vi "2D barcode scanning.vi"() -> ()   [LabVIEW 2015]
panel:
  in  "Find Max and Min":bool
  out "Optical Angle Waveform Graph":dynamicdata(graph)
  out "PSD Waveform Graph":dynamicdata(graph)
  out "Photodiode Waveform Graph":dynamicdata(graph)
  out "XY Graph":cluster{"Y":dbl[], "Y":dbl[]}[](graph)
  out "Offset Voltage":dbl
  out "Optical Angle":dynamicdata(graph)
  out "Min. Volt":dbl
  out "Max. Volt":dbl
  out "PSD Voltage":dbl format="%_15g"
  out "PSD (voltage)":dynamicdata(graph)
  out "Photodiode Waveform Chart (V)":dynamicdata(graph)
  out "Photodiode":dbl
  in  "stop (F)":bool
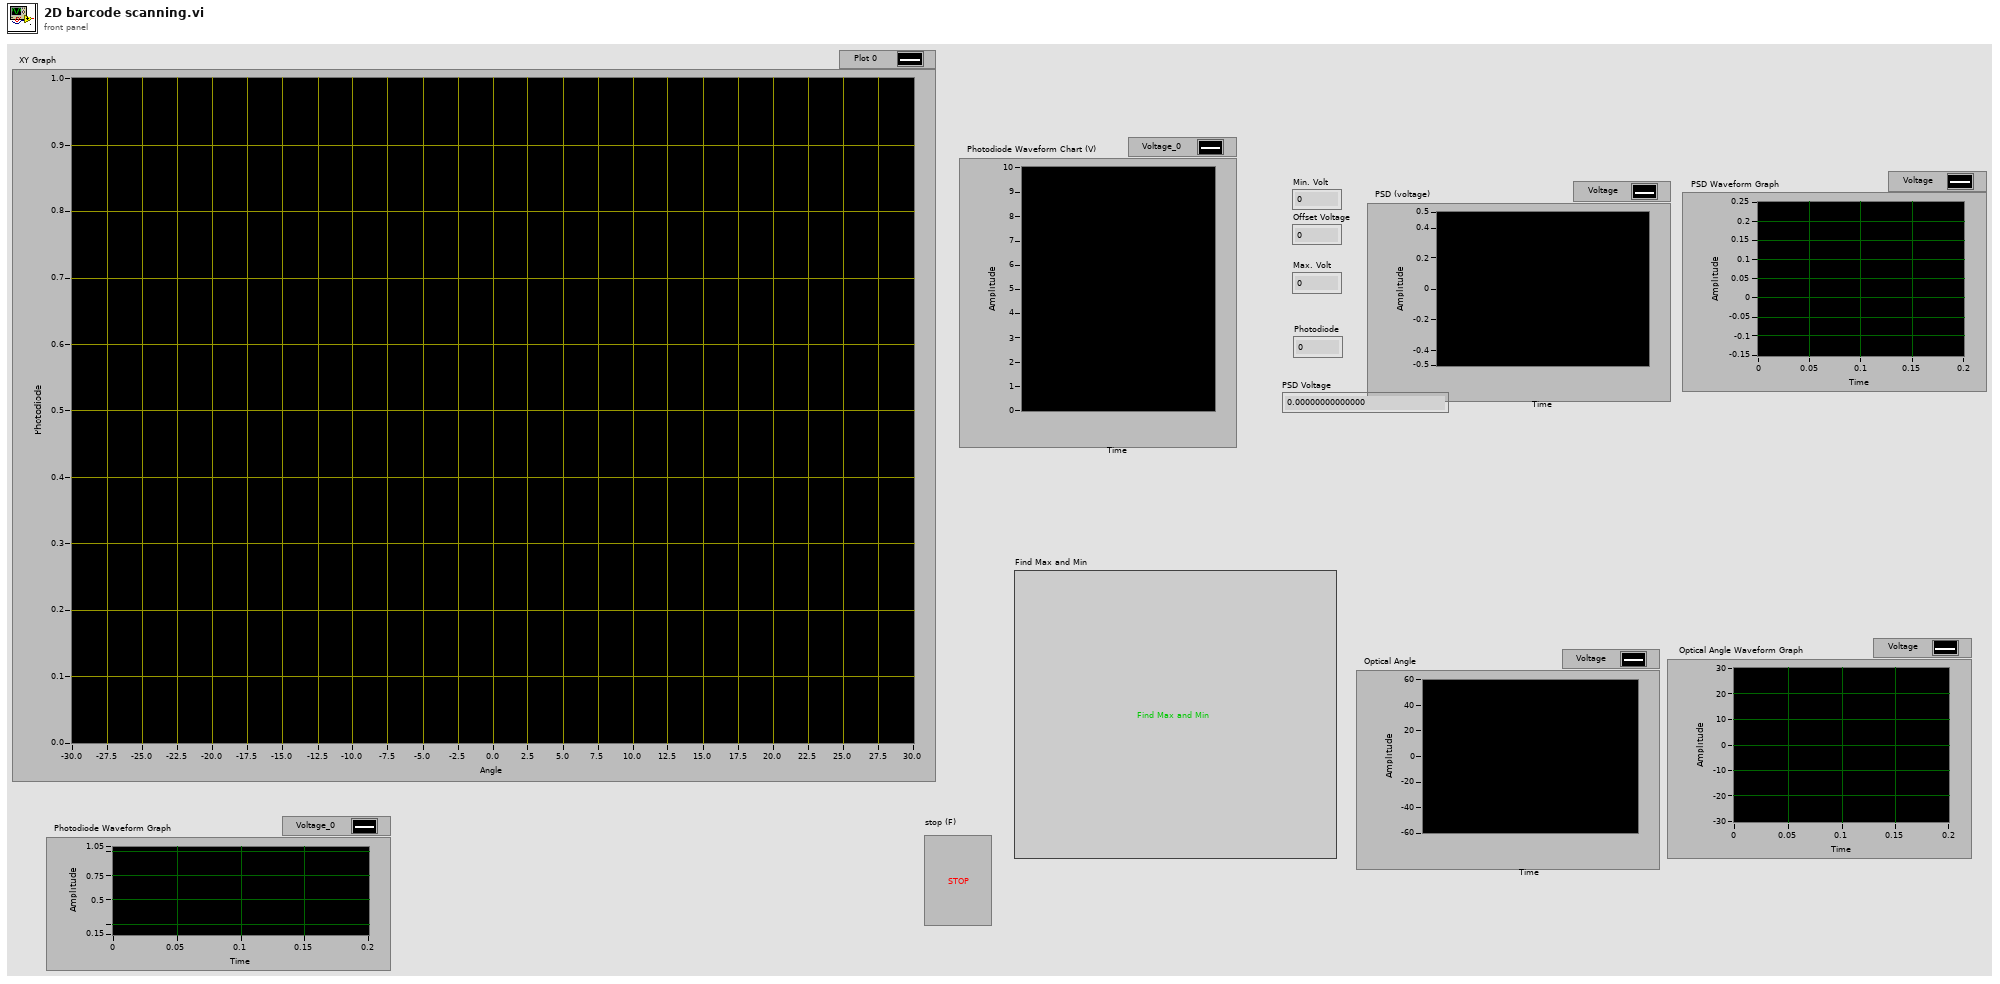
[diagram p1: front panel]
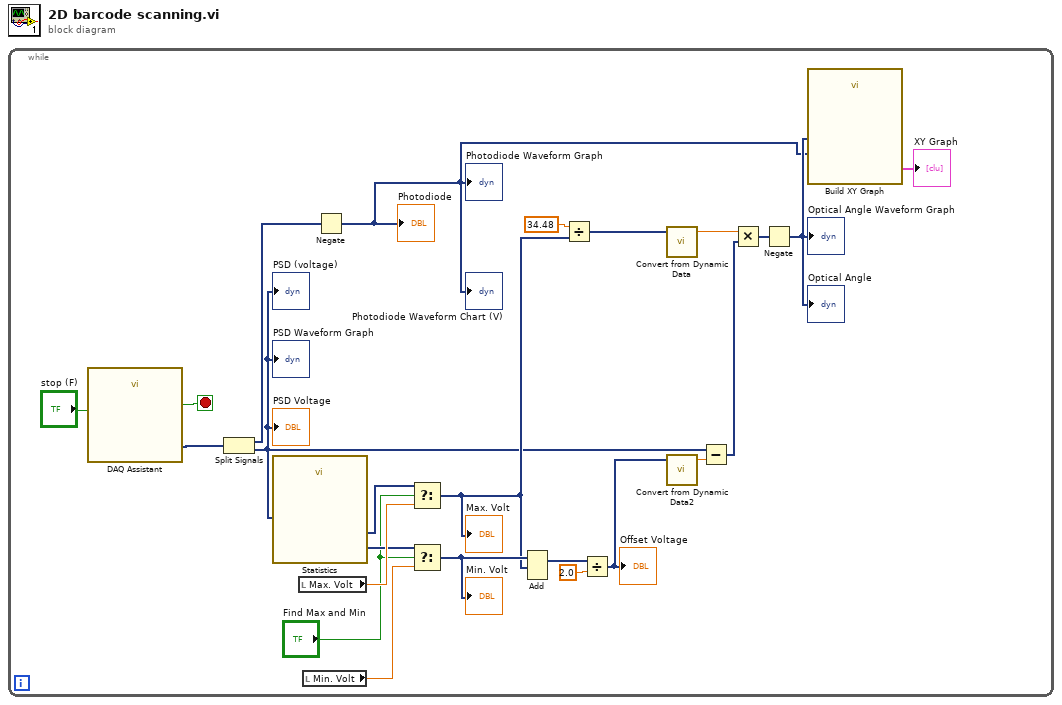
[diagram p0: block diagram]
diagram:
  n1 = while {
    stop <- w23 stop-if-true
    n2 = call "DAQ Assistant"("stop (F)"="stop (F)") -> ("data"=w22:dynamicdata, "stopped"=w23:bool)  [unwired: 15 in, 2 out]
    n3 = Split Signals(w22) -> (w5:dynamicdata, w3:dynamicdata)  [unwired: 2 in]
    "PSD (voltage)" <- w3
    "PSD Voltage" <- w3
    "PSD Waveform Graph" <- w3
    n4 = call "Statistics"("Signals"=w3) -> ("Minimum"=w15:dynamicdata, "Maximum"=w17:dynamicdata)  [unwired: 24 in, 1 out]
    n5 = local read "Max. Volt"() -> (w20:dbl)
    n6 = local read "Min. Volt"() -> (w16:dbl)
    n7 = Negate(x=w5) -> (-x=w4:dynamicdata)
    "Photodiode" <- w4
    "Photodiode Waveform Chart (V)" <- w4
    "Photodiode Waveform Graph" <- w4
    n8 = Select(t=w17, s="Find Max and Min", f=w20) -> (s? t:f=w13:dynamicdata)
    "Max. Volt" <- w13
    n9 = Select(t=w15, s="Find Max and Min", f=w16) -> (s? t:f=w14:dynamicdata)
    "Min. Volt" <- w14
    n10 = Add(1:w13, 2:w14) -> (0:w12:dynamicdata)  [unwired: 1 in, 1 out]
    n11 = Divide(x=34.48, y=w13) -> (x/y=w18:dynamicdata)
    n12 = Divide(x=w12, y=2.0) -> (x/y=w10:dynamicdata)
    "Offset Voltage" <- w10
    n13 = call "Convert from Dynamic Data"("Dynamic Data Type"=w18) -> ("Scalar"=w19:dbl)  [unwired: 3 in]
    n14 = call "Convert from Dynamic Data2"("Dynamic Data Type"=w10) -> ("Scalar"=w9:dbl)  [unwired: 3 in]
    n15 = Subtract(x=w3, y=w9) -> (x-y=w2:dynamicdata)
    n16 = Multiply(x=w19, y=w2) -> (x*y=w1:dynamicdata)
    n17 = Negate(x=w1) -> (-x=w7:dynamicdata)
    "Optical Angle" <- w7
    "Optical Angle Waveform Graph" <- w7
    n18 = call "Build XY Graph"("Y Input"=w4, "X Input"=w7) -> ("XY Graph"=→"XY Graph":cluster{"X":dbl[], "Y":dbl[]}[])  [unwired: 8 in, 1 out]
  }
